vi "Configure User Trigger Delay.vi"(6 "User Defined Delay (0 s)":dbl, 7 "User (1: USER1)":i32(ring)=1 items=["USER1"=1, "USER2"=2, "USER3"=3, "USER4"=4, "USER5"=5], 8 "error in (no error)":errorcluster, 9 "Channel List(\"\")":string, 10 "Function (0: Voltage DC)":i32(ring) items=[" Voltage DC", "Voltage AC", "Current DC", "Current AC", "Resistance", "4-wire Resistance", "Diode", "Capacitance", "Temperature", "Continuity", "Frequency", "Period", "Voltage Ratio", "Digitize Voltage", "Digitize Current"], 11 "VISA resource name":refnum<visa-resource-name>) -> (0 "error out":errorcluster, 3 "VISA resource name out":refnum<visa-resource-name>)   [LabVIEW 2023, in "Keithley DMM6500 DAQ6500 Series.lvlib"]
doc: "Configures a user-defined trigger delay that you can use in the trigger model."
uses:
  <instrlib>/Keithley DMM6500 DAQ6500 Series/Keithley DMM6500 DAQ6500 Series.lvlib
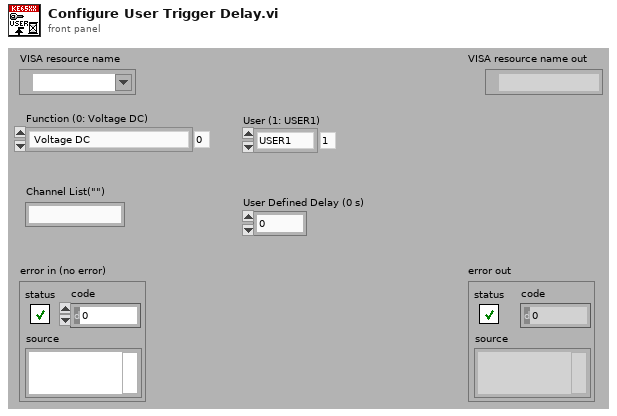
[diagram p1: front panel]
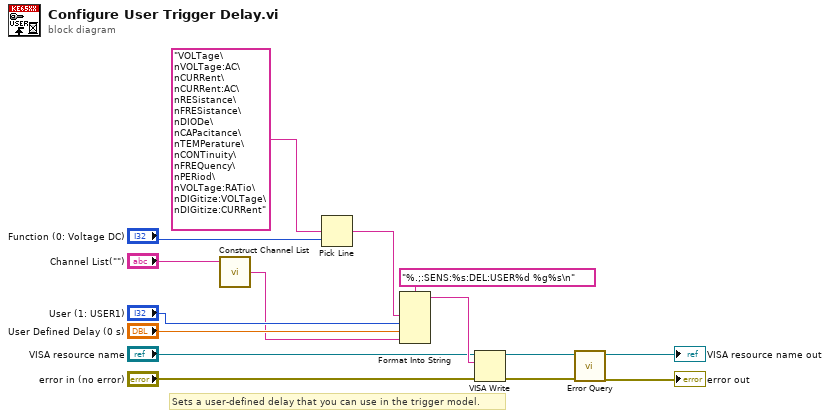
[diagram p0: block diagram]
diagram:
  # "Sets a user-defined delay that you can use in the trigger model."
  n1 = call <instrlib>:"Construct Channel List.vi"("Channel List"="Channel List(\"\")") -> ("Channel List String"=w3:string)  [unwired: 2 in]
  n2 = Pick Line(multi-line string="VOLTage\nVOLTage:AC\nCURRent\nCURRent:AC\nRESistance\nFRESistance\nDIODe\nCAPacitance\nTEMPerature\nCONTinuity\nFREQuency\nPERiod\nVOLTage:RATio\nDIGitize:VOLTage\nDIGitize:CURRent", line index="Function (0: Voltage DC)") -> (output string=w2:string)  [unwired: 1 in]
  n3 = Format Into String(format string="%.;:SENS:%s:DEL:USER%d %g%s\n", w2, "User (1: USER1)", "User Defined Delay (0 s)", w3) -> (resulting string=w13:string)  [unwired: 2 in, 1 out]
  n4 = VISA Write(VISA resource name="VISA resource name", write buffer=w13, error in (no error)="error in (no error)") -> (VISA resource name out=w10:refnum<visa-resource-name>, error out=w9:errorcluster)  [unwired: 1 out]
  n5 = call <instrlib>:"Error Query.vi"("error in (no error)"=w9, "VISA resource name"=w10) -> ("error out"=→"error out":errorcluster, "VISA resource name out"=→"VISA resource name out":refnum<visa-resource-name>)  [unwired: 6 in, 2 out]
